vi "prepractica 2.vi"() -> ()   [LabVIEW 2015]
panel:
  out "Resultado:":dbl
  in  "Factorial de:":dbl
  in  "Comprobar":bool
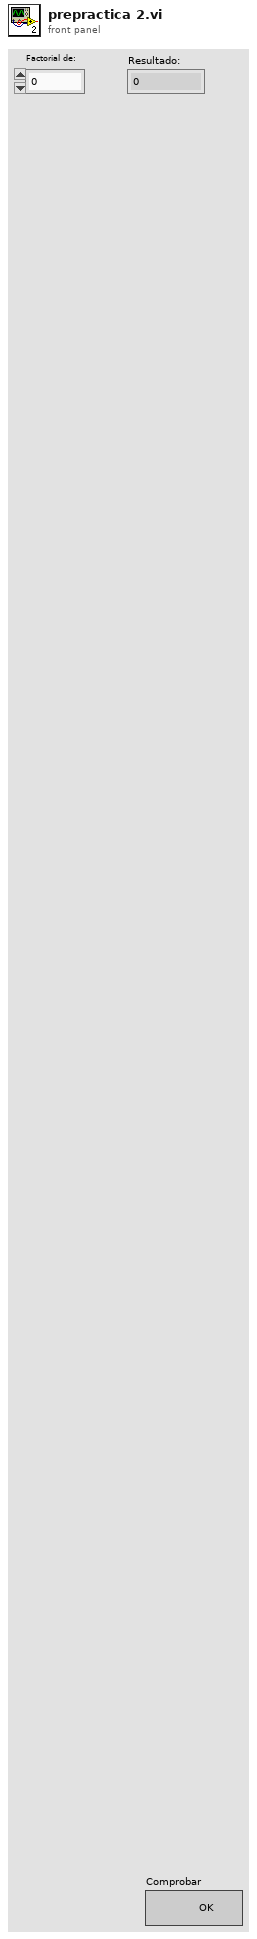
[diagram p1: front panel]
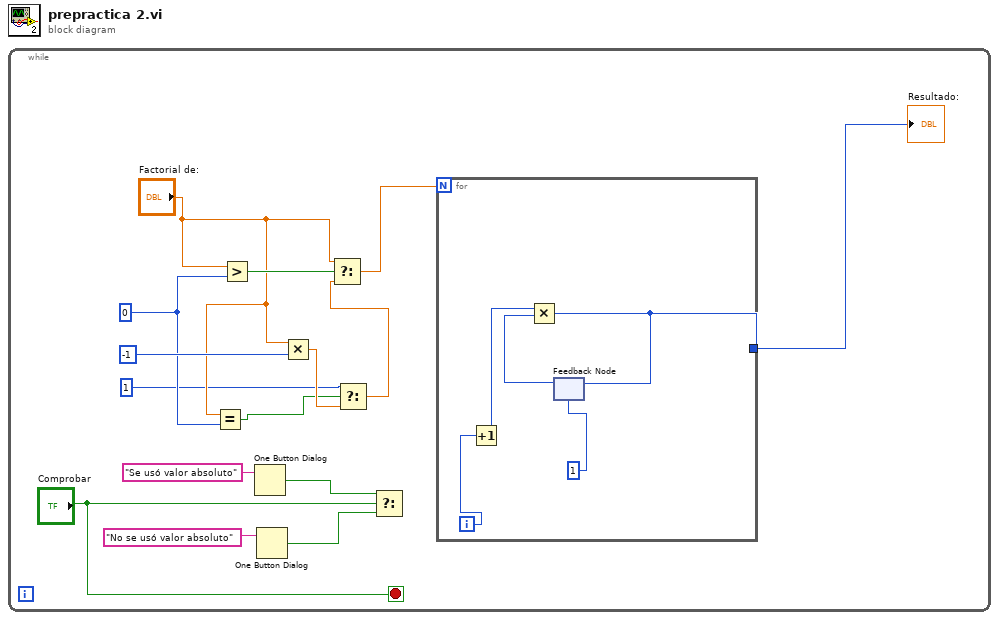
[diagram p0: block diagram]
diagram:
  n1 = while {
    stop <- "Comprobar" stop-if-true
    w3 = 0
    n2 = Equal?(x="Factorial de:", y=w3) -> (x = y?=w2:bool)
    n3 = Greater?(x="Factorial de:", y=w3) -> (0:w5:bool)
    n4 = One Button Dialog(message="Se usó valor absoluto" ("button name (\"OK\")")) -> (true=w13:bool)  [unwired: 1 in]
    n5 = One Button Dialog(message="No se usó valor absoluto" ("button name (\"OK\")")) -> (true=w12:bool)  [unwired: 1 in]
    n6 = Multiply(x="Factorial de:", y=-1) -> (x*y=w7:dbl)
    n7 = Select(t=1, s=w2, f=w7) -> (s? t:f=w6:dbl)
    n8 = Select(t="Factorial de:", s=w5, f=w6) -> (s? t:f=w8:dbl)
    n9 = Select(t=w13, s="Comprobar", f=w12) -> ()  [unwired: 1 out]
    n10 = for {
      N: w8 -> [_]
      tunnel: [w16] -> w10
      i -> [w20]
      n11 = Increment(x=w20) -> (x+1=w19:i32)
      n12 = feedback #1(1) -> (w17:i32)
      n13 = Multiply(x=w19, y=w17) -> (x*y=w16:i32)
      n14 = feedback-in #1(w16) -> ()
    }
    "Resultado:" <- w10
  }
